vi "current test.vi"() -> ()   [LabVIEW 2014]
panel:
  out "voltage (V)":dbl
  out "all currents (A)":dbl[](array[numeric])
  out "Power (W)":dbl
  out "Energy (J)":dbl
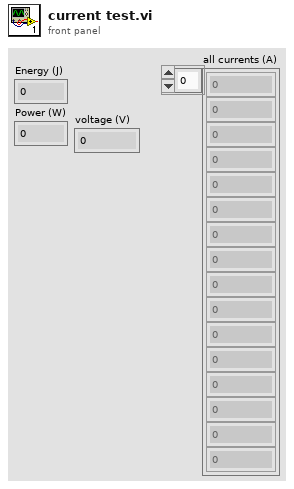
[diagram p1: front panel]
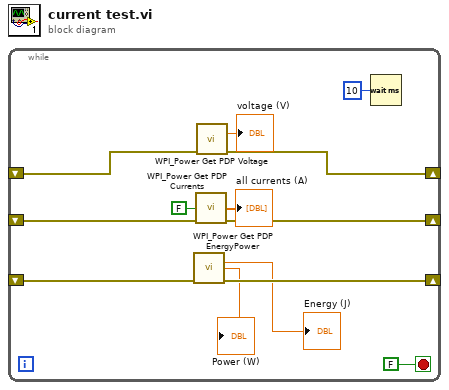
[diagram p0: block diagram]
diagram:
  n1 = while {
    shift-right: [w12] -> _
    shift-left: _ -> [w11]
    shift-right: [w9] -> _
    shift-left: _ -> [w8]
    shift-right: [w10] -> _
    shift-left: _ -> [w7]
    stop <- FALSE stop-if-true
    n2 = call <vilib>:"WPI_Power Get PDP EnergyPower.vi"("error in"=w8) -> ("Energy (J)"=→"Energy (J)":dbl, "Power (W)"=→"Power (W)":dbl, "error out"=w9:errorcluster)  [unwired: 12 in]
    n3 = call <vilib>:"WPI_Power Get PDP Currents.vi"("Tare Currents?"=FALSE, "error in"=w7) -> ("all currents (A)"=→"all currents (A)":dbl[], "error out"=w10:errorcluster)  [unwired: 11 in, 1 out]
    n4 = call <vilib>:"WPI_Power Get PDP Voltage.vi"("error in"=w11) -> ("voltage (V)"=→"voltage (V)":dbl, "error out"=w12:errorcluster)  [unwired: 13 in]
    n5 = Wait (ms)(milliseconds to wait=u32 10) -> ()  [unwired: 1 out]
  }
